vi "Condition Type.vi"(11 "Time Condition Config in":refnum<class "Time Condition Config.lvclass">) -> (2 "Condition Type":string)   [LabVIEW 2020, in "VolatusSeqConfig.lvlib" / "Time Condition Config.lvclass"]
uses:
  Time Condition Config.lvclass
  Time Condition Config.lvclass/Time Condition Config.ctl
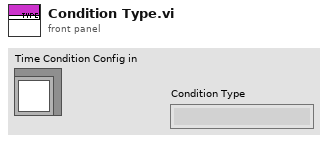
[diagram p1: front panel]
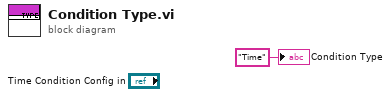
[diagram p0: block diagram]
diagram:
  "Condition Type" <- "Time" ("Condition Type")
